vi "writeVideo.vi"(7 "Image pointer recycler queue":refnum<queue>, 8 "error in (no error)":errorcluster, 9 "Trigger timestamps":T3, 10 "Video queue":refnum<queue>, 11 "AVI file reference in":T2) -> (0 "error out":errorcluster, 1 "timeState":T1(ring), 2 "Writing video?":bool, 3 "AVI file reference out":T2)   [LabVIEW 2017]
doc: "If video is present in queue, write it to disk."
uses:
  <vilib>/vision/Image Controls.llb/IMAQ Image.ctl
  <vilib>/vision/Avi.llb/IMAQ AVI2 Refnum.ctl
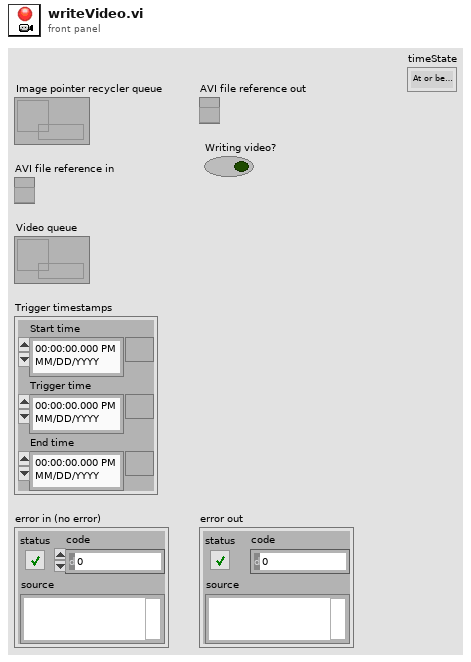
[diagram p1: front panel]
types:
  T1 = enum16{"At or before start", "In range", "At or after end"}
  T2 = typedef "IMAQ AVI2 Refnum.ctl" = refnum<k20>
  T3 = cluster{"Start time":timestamp, "Trigger time":timestamp, "End time":timestamp}
  T4 = typedef "IMAQ Image.ctl" = refnum<image>
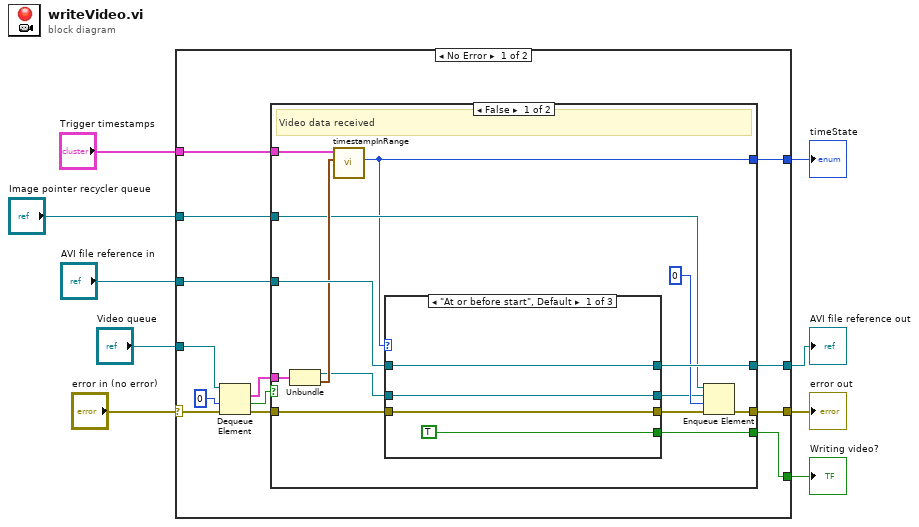
[diagram p0: block diagram]
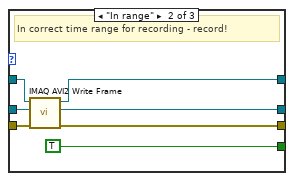
[diagram p2: hidden frame]
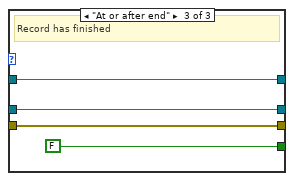
[diagram p3: hidden frame]
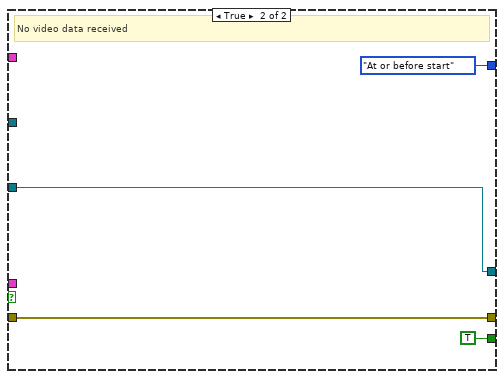
[diagram p4: hidden frame]
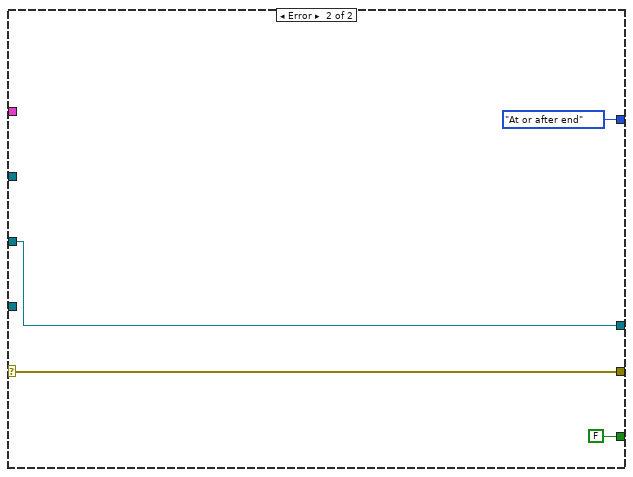
[diagram p5: hidden frame]
diagram:
  n1 = case shown="No Error" "error in (no error)" {
    selector: "error in (no error)" -> [w15 w57]
    tunnel: [w22 FALSE ("Write to file")] -> w9
    tunnel: [w20 w57] -> w8
    tunnel: [w16 w58] -> w7
    tunnel: "AVI file reference in" -> [w14 w58]
    tunnel: "Image pointer recycler queue" -> [w13 _]
    tunnel: "Trigger timestamps" -> [w12 _]
    tunnel: "Video queue" -> [w11 _]
    tunnel: [w10 T1."At or after end" ("timeState")] -> w1
    frame No Error {
      n2 = Dequeue Element(queue=w11, timeout in ms (-1)=0, error in (no error)=w15) -> (element=w18:cluster{"Image Out":T4, timestamp}, timed out?=w21:bool, error out=w17:errorcluster)  [unwired: 1 out]
      n3 = case shown="False" w21 {
        tunnel: [w36 w54] -> w16
        tunnel: w14 -> [w35 w54]
        tunnel: w17 -> [w34 w53]
        tunnel: w18 -> [w33 _]
        tunnel: w13 -> [w31 _]
        tunnel: [w26 TRUE ("Write to file")] -> w22
        tunnel: [w25 w53] -> w20
        tunnel: w12 -> [w24 _]
        tunnel: [w23 T1."At or before start" ("timeState")] -> w10
        frame False {
          # "Video data received"
          n4 = Unbundle(w33) -> ("Image Out"=w28:T4, w32:timestamp)
          n5 = call "timestampInRange.vi"("Time Stamp"=w32, "Start and end times"=w24) -> ("timeState"=w23:T1)  [unwired: 9 in]
          n6 = case shown="\"At or before start\", Default" w23 {
            tunnel: w34 -> [w38 w44 w51]
            tunnel: w28 -> [w39 w41 w49]
            tunnel: [w40 w47 w50] -> w36
            tunnel: [w38 w43 w51] -> w30
            tunnel: w35 -> [w40 w46 w50]
            tunnel: [w39 w45 w49] -> w27
            tunnel: [TRUE ("Write to file") TRUE FALSE ("Write to file")] -> w26
            frame "At or before start", Default {
            }
            frame "In range" {
              # "In correct time range for recording - record!"
              n7 = call "IMAQ AVI2 Write Frame"("error in (no error)"=w44, "Image"=w41, "AVI Refnum"=w46) -> ("error out"=w43:errorcluster, "Image Out (duplicate)"=w45:T4, "AVI Refnum (duplicate)"=w47:T2)  [unwired: 6 in]
            }
            frame "At or after end" {
              # "Record has finished"
            }
          }
          n8 = Enqueue Element(queue=w31, element=w27, timeout in ms (-1)=0, error in (no error)=w30) -> (error out=w25:errorcluster)  [unwired: 2 out]
        }
        frame True {
          # "No video data received"
        }
      }
    }
    frame Error {
    }
  }
  "Writing video?" <- w9
  "error out" <- w8
  "AVI file reference out" <- w7
  "timeState" <- w1
